vi "BuildVICallChain.vi"() -> (0 "CallChain":string)   [LabVIEW 2018]
doc: "This VI is used to generate a string that defines the chain of calling VIs from the top-level down to the VI in which this subVI resides.\n\nCopyright © 2011 Epimedia, Inc. All Rights Reserved.\n\nThe Epimedia Application Library is Copyright © 2009-2011 Epimedia, Inc. \nAll Rights Reserved. Used under license."
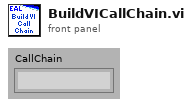
[diagram p1: front panel]
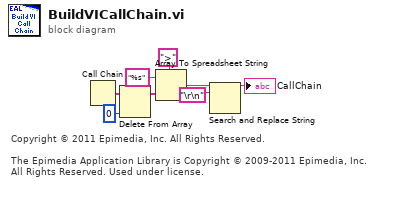
[diagram p0: block diagram]
diagram:
  # "Copyright © 2011 Epimedia, Inc. All Rights Reserved.\n\nThe Epimedia Application Library is Copyright © 2009-2011 Epimedia, Inc. \nAll Rights Reserved. Used under license."
  n1 = Call Chain() -> (call chain=w3:string[])
  n2 = Delete From Array(array=w3, index=0) -> (array with subset deleted=w1:string[])  [unwired: 1 in, 1 out]
  n3 = Array To Spreadsheet String(delimiter (Tab)=">", array=w1, 3:"%s" ("format string")) -> (spreadsheet string=w6:string)
  n4 = Search and Replace String(input string=w6, search string="\r\n") -> (result string=→"CallChain":string)  [unwired: 1 in, 8 out]
